vi "SQL_param_alarm_update.vi"(11 "表格控件":string[][](table)=[["陪试轴承润滑单元_出油温度", "0", "200", "1"], ["实验轴承润滑单元_外壳振动", "0", "100", "1"], ["实验轴承润滑单元_轴承外圈温度", "0", "100", "1"], ["实验轴承润滑单元_声发射", "0", "100", "1"], ["实验轴承润滑单元_出油温度", "0", "100", "1"], ["实验轴承润滑单元_摩擦力矩1", "0", "100", "1"], ["实验轴承润滑单元_摩擦力矩2", "0", "100", "1"], ["加载单元_径向油缸力", "0", "100", "1"], ["加载单元_轴向油缸力", "0", "100", "1"], ["主轴监测单元_4个2X/2Y位移", "0", "100", "1"], ["主轴监测单元_1个径向位移", "0", "100", "1"], ["主轴监测单元_1个转速", "0", "100", "1"]]) -> (3 "error out":errorcluster)   [LabVIEW 2014]
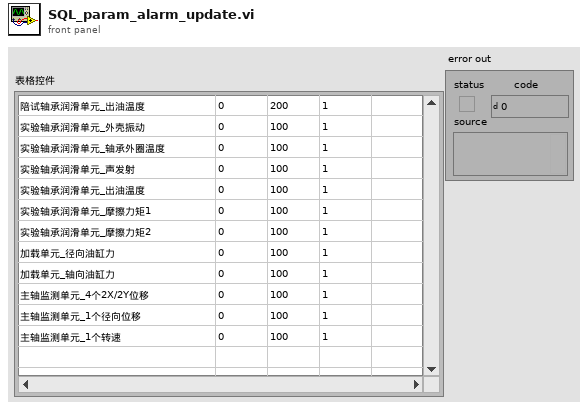
[diagram p1: front panel]
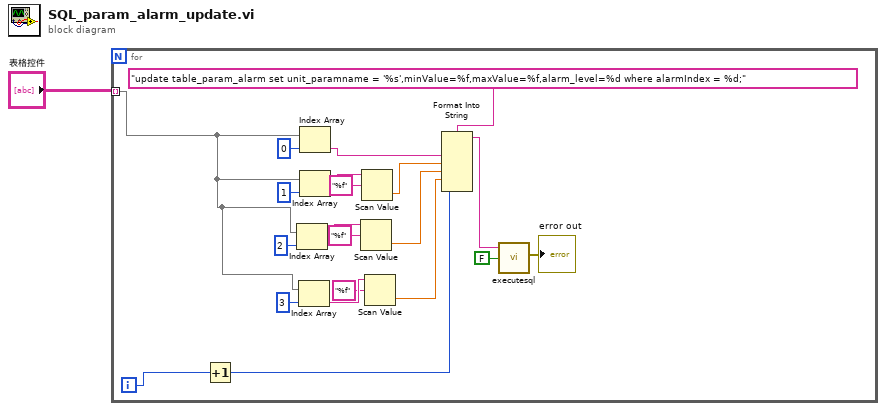
[diagram p0: block diagram]
diagram:
  n1 = for {
    tunnel: "表格控件" -> [w8] mode=indexing
    i -> [w4]
    n2 = Increment(x=w4) -> (x+1=w3:i32)
    n3 = Index Array(array=w8, index=2 ("索引")) -> (element=w13:string)
    n4 = Index Array(array=w8, index=3 ("索引")) -> (element=w10:string)
    n5 = Index Array(array=w8, index=0 ("索引")) -> (element=w20:string)
    n6 = Index Array(array=w8, index=1 ("索引")) -> (element=w18:string)
    n7 = Scan Value(string=w13, format string="%f" ("格式字符串")) -> (value=w12:dbl)  [unwired: 1 in, 1 out]
    n8 = Scan Value(string=w18, format string="%f" ("格式字符串")) -> (value=w17:dbl)  [unwired: 1 in, 1 out]
    n9 = Scan Value(string=w10, format string="%f" ("格式字符串")) -> (value=w9:dbl)  [unwired: 1 in, 1 out]
    n10 = Format Into String(format string="update table_param_alarm set unit_paramname = '%s',minValue=%f,maxValue=%f,alarm_level=%d where alarmIndex = %d;", w20, w17, w12, w9, w3) -> (resulting string=w16:string)  [unwired: 2 in, 1 out]
    n11 = call "executesql.vi"("Return Data (T)"=FALSE, "Command Text"=w16) -> ("error out"=→"error out":errorcluster)  [unwired: 5 in, 1 out]
  }
